vi "Data Files Control.vi"(7 "Comm":enum16{"Get", "Put"}(ring), 8 "에러 입력":errorcluster caption="에러 입력(에러 없음)", 11 "Slide 입력":refnum<vi>) -> (0 "에러 출력":errorcluster)   [LabVIEW 2020]
uses:
  Controls/Cmd_File path.ctl
  <vilib>/FTP/NI_FTP.lvlib
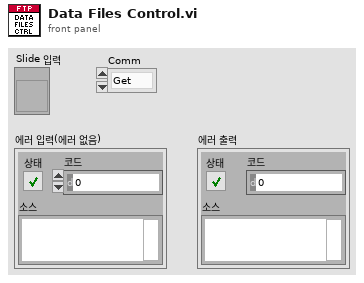
[diagram p1: front panel]
types:
  T1 = typedef "Cmd_File path.ctl" = enum16{"에러로그", "데이터파일경로", "성적서원본", "지난성적서", "Data Files", "경로생성", "Updater", "Template", "설정파일경로", "FTP Upload", "Update 경로", "어플리케이션"}
  T2 = typedef "NI_FTP.lvlib/FTP Session.ctl" = refnum<k5>
  T3 = cluster{"date":string, "byte":string, "name":string}[]
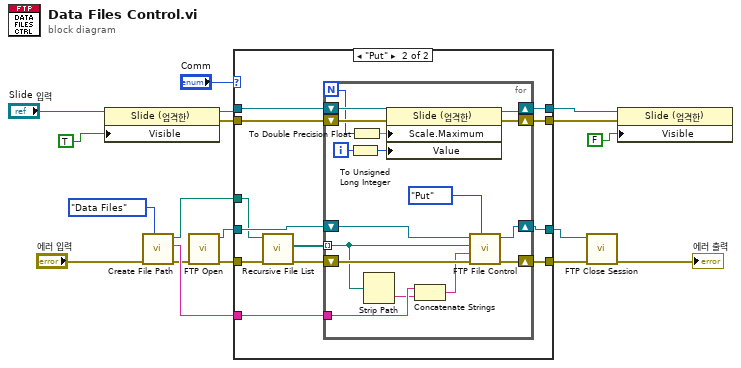
[diagram p0: block diagram]
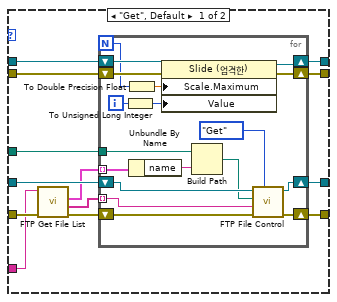
[diagram p2: hidden frame]
diagram:
  n1 = property class="Slide (엄격한)"(reference="Slide 입력", "Visible"=TRUE ("보이기")) -> (reference out=w11:refnum<vi>, error out=w12:errorcluster)  [unwired: 1 in]
  n2 = call "Create File Path.vi"("항목"=Cmd_File_path."Data Files", "에러 입력"="에러 입력") -> ("error out"=w1:errorcluster, "문자열 out"=w3:string, "파일경로"=w2:path)  [unwired: 6 in, 1 out]
  n3 = call "FTP Open.vi"("에러 입력(에러 없음)"=w1) -> ("에러 출력"=w7:errorcluster, "TCP 네트워크 연결 출력"=w15:T2)  [unwired: 9 in]
  n4 = case shown="\"Put\"" "Comm" {
    tunnel: [w27 w61] -> w17
    tunnel: [w26 w60] -> w16
    tunnel: w15 -> [w25 w59]
    tunnel: w2 -> [w19 w58]
    tunnel: w3 -> [w22 w56]
    tunnel: w12 -> [w29 w55]
    tunnel: w11 -> [w30 w54]
    tunnel: [w28 w53] -> w9
    tunnel: [w31 w52] -> w8
    tunnel: w7 -> [w24 w51]
    frame "Get", Default {
      n5 = call "FTP Get File List.vi"("에러 입력(에러 없음)"=w24, "remote path"=w22) -> ("에러 출력"=w23:errorcluster, "remote File path"=w20:string[], "File List"=w21:T3)  [unwired: 6 in, 1 out]
      n6 = for {
        N -> [w38]
        shift-right: [w47] -> w27
        shift-left: w23 -> [w49]
        shift-right: [w46] -> w26
        shift-left: w25 -> [w48]
        tunnel: w20 -> [w33] mode=indexing
        tunnel: w19 -> [w45]
        tunnel: w21 -> [w44] mode=indexing
        shift-right: [w35] -> w31
        shift-left: w30 -> [w41]
        shift-right: [w36] -> w28
        shift-left: w29 -> [w42]
        i -> [w40]
        n7 = To Unsigned Long Integer(number=w40) -> (unsigned 32bit integer=w39:u32)
        n8 = To Double Precision Float(number=w38) -> (double precision float=w37:dbl)
        n9 = Unbundle By Name(w44) -> ("name"=w43:string)
        n10 = property class="Slide (엄격한)"(reference=w41, error in=w42, "Scale.Maximum"=w37, "Value"=w39) -> (reference out=w35:refnum<vi>, error out=w36:errorcluster)
        n11 = Build Path(base path=w45, name or relative path=w43) -> (appended path=w32:path)
        n12 = call "FTP File Control.vi"("Comm"=enum16{"Get", "Put"}."Get", "에러 입력"=w49, "원격경로"=w33, "로컬경로"=w32, "TCP 네트워크 연결 입력"=w48) -> ("에러 출력"=w47:errorcluster, "TCP 네트워크 연결 출력"=w46:T2)  [unwired: 2 in, 3 out]
      }
    }
    frame "Put" {
      n13 = call <vilib>:"Recursive File List.vi"("error in (no error)"=w51, "Folder Path"=w58) -> ("error out"=w50:errorcluster, "All Files in Dir"=w57:path[])  [unwired: 5 in, 3 out]
      n14 = for {
        N -> [w68]
        shift-right: [w78] -> w61
        shift-left: w50 -> [w77]
        shift-right: [w75] -> w60
        shift-left: w59 -> [w76]
        tunnel: w57 -> [w62] mode=indexing
        tunnel: w56 -> [w74]
        shift-right: [w65] -> w52
        shift-left: w54 -> [w69]
        shift-right: [w66] -> w53
        shift-left: w55 -> [w70]
        i -> [w67]
        n15 = To Unsigned Long Integer(number=w67) -> (unsigned 32bit integer=w72:u32)
        n16 = To Double Precision Float(number=w68) -> (double precision float=w71:dbl)
        n17 = Strip Path(path=w62) -> (name=w73:string)  [unwired: 1 out]
        n18 = property class="Slide (엄격한)"(reference=w69, error in=w70, "Scale.Maximum"=w71, "Value"=w72) -> (reference out=w65:refnum<vi>, error out=w66:errorcluster)
        n19 = Concatenate Strings(w74, w73) -> (w63:string)
        n20 = call "FTP File Control.vi"("Comm"=enum16{"Get", "Put"}."Put", "에러 입력"=w77, "원격경로"=w63, "로컬경로"=w62, "TCP 네트워크 연결 입력"=w76) -> ("에러 출력"=w78:errorcluster, "TCP 네트워크 연결 출력"=w75:T2)  [unwired: 2 in, 3 out]
      }
    }
  }
  n21 = call <vilib>:"FTP Close Session.vi"("error in (no error)"=w17, "ftp session"=w16) -> ("error out"=→"에러 출력":errorcluster)  [unwired: 6 in, 3 out]
  n22 = property class="Slide (엄격한)"(reference=w8, error in=w9, "Visible"=FALSE ("보이기")) -> ()  [unwired: 2 out]
